vi "CreateRoomWalls.vi"(7 "WallID":T1, 8 "error in (no error)":errorcluster, 10 "DirectionsList":T3[](array[typedef]), 11 "MazeGame":refnum<class "MazeGame.lvclass">) -> (0 "error out":errorcluster, 2 "RoomWallsList":T2[](array[typedef]), 3 "MazeGame":refnum<class "MazeGame.lvclass">)   [LabVIEW 2020, in "FactoryMethod.lvlib" / "ParameterizedFactoryMethod.lvlib" / "MazeGame.lvclass"]
uses:
  MazeGame.lvclass
  GoFcommonClasses/Direction.ctl
  NoParametrizedFactoryMethod/MazeGame/Private/TypeDef/RoomElement.ctl
  GoFcommonClasses/MazeSite/MazeSite.lvclass
  API/TypeDef/WallID.ctl
  GoFcommonClasses/ConcreteMazeSite/Wall/Wall.lvclass
  E:/Francesco/GitHub/Design-Patterns-GoF_-_NI-LV/Creational/GoFcommonClasses/MazeSite/MazeSite.lvclass
  GoFcommonClasses/ConcreteMazeSite/Room/Room.lvclass
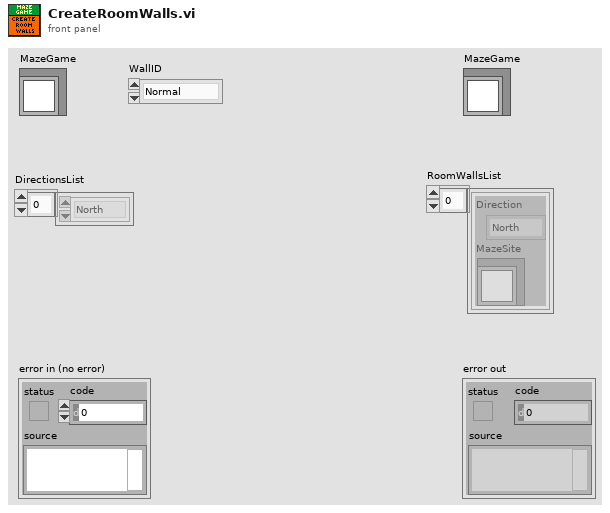
[diagram p1: front panel]
types:
  T1 = typedef "FactoryMethod.lvlib/ParameterizedFactoryMethod.lvlib/MazeGame.lvclass/WallID.ctl" = enum8{"Normal", "Bombed"}
  T2 = typedef "Room.lvclass/RoomElement.ctl" = cluster{"Direction":T3, "MazeSite":refnum<class "MazeSite.lvclass">}
  T3 = typedef "Direction.ctl" = enum32{"North", "South", "East", "West"}
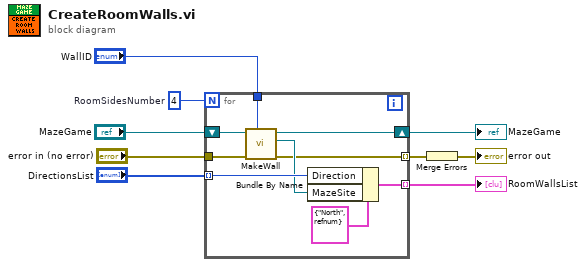
[diagram p0: block diagram]
diagram:
  w4 = 4  # RoomSidesNumber
  n1 = for {
    N: w4 -> [_]
    tunnel: "DirectionsList" -> [w18] mode=indexing
    tunnel: [w17] -> w6 mode=indexing
    tunnel: "error in (no error)" -> [w15]
    tunnel: [w14] -> w7 mode=indexing
    shift-right: [w11] -> w2
    shift-left: "MazeGame" -> [w12]
    tunnel: "WallID" -> [w10]
    n2 = call-dynamic "MakeWall.vi"("WallID"=w10, "error in (no error)"=w15, "MazeGame"=w12) -> ("error out"=w14:errorcluster, "Wall"=w16:refnum<class "Wall.lvclass">, "MazeGame"=w11:refnum<class "MazeGame.lvclass">)  [unwired: 6 in]
    n3 = Bundle By Name(cluster=T2 {"Direction"=enum."North", "MazeSite"=refnum} ("RoomElement"), "Direction"=w18, "MazeSite"=w16) -> (w17:T2)
  }
  "MazeGame" <- w2
  "RoomWallsList" <- w6
  n4 = Merge Errors(w7) -> (→"error out":errorcluster)
